vi "Unequal_Safe_2dBOOL.vi"(5 "x":bool[][](array[boolean]), 9 "y":bool[][](array[boolean])) -> (8 "Diff?":bool, 14 "Diff? array":bool[][](array[boolean]))   [LabVIEW 2013]
doc: "Assesses x not equal to y?, up to length of x. The output 'which diff?' always matches the length of x. Additionally, 'diff?' is provided for convenience as the array-OR for a simple boolean indicating at lease one difference."
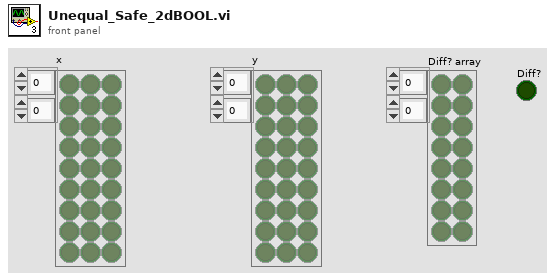
[diagram p1: front panel]
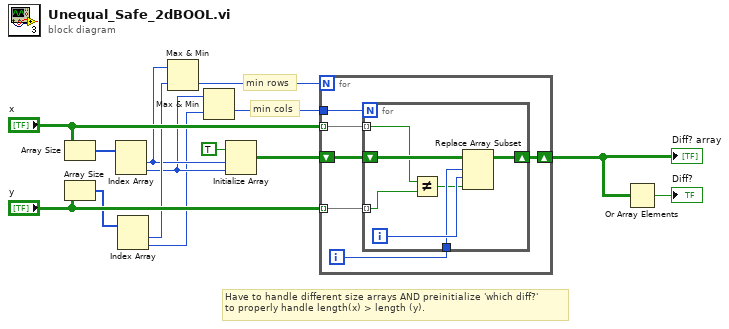
[diagram p0: block diagram]
diagram:
  # "min cols"
  # "Have to handle different size arrays AND preinitialize 'which diff?'\nto properly handle length(x) > length (y)."
  # "min rows"
  n1 = Array Size(array="x") -> (size(s)=w8:i32[])
  n2 = Array Size(array="y") -> (size(s)=w7:i32[])
  n3 = Index Array(array=w8) -> (element #1=w5:i32, element #2=w3:i32)  [unwired: 2 in]
  n4 = Index Array(array=w7) -> (element #1=w6:i32, element #2=w2:i32)  [unwired: 2 in]
  n5 = Max & Min(x=w5, y=w6) -> (min(x,y)=w4:i32)  [unwired: 1 out]
  n6 = Max & Min(x=w3, y=w2) -> (min(x,y)=w1:i32)  [unwired: 1 out]
  n7 = Initialize Array(TRUE, w5, w3) -> (w9:bool[][])
  n8 = for {
    N: w4 -> [_]
    tunnel: "x" -> [w20] mode=indexing
    tunnel: "y" -> [w19] mode=indexing
    shift-right: [w18] -> w12
    shift-left: w9 -> [w17]
    tunnel: w1 -> [w15]
    i -> [w16]
    n9 = for {
      N: w15 -> [_]
      tunnel: w19 -> [w24] mode=indexing
      tunnel: w20 -> [w25] mode=indexing
      tunnel: w16 -> [w22]
      shift-right: [w26] -> w18
      shift-left: w17 -> [w27]
      i -> [w23]
      n10 = Not Equal?(x=w25, y=w24) -> (x != y?=w21:bool)
      n11 = Replace Array Subset(array=w27, new element=w21, index (row)=w22, index (col)=w23) -> (w26:bool[][])
    }
  }
  "Diff? array" <- w12
  n12 = Or Array Elements(Boolean array=w12) -> (logical OR=→"Diff?":bool)
